vi "Get Board Information.vi"(8 "error in (no error)":errorcluster) -> (0 "error out":errorcluster, 3 "Board Information":string)   [LabVIEW 2021, in "Utilities.lvlib"]
doc: "Returns information of the application board that you connect to the NI ELVIS III workstation, such as the board ID and board status."
uses:
  <vilib>/myRIO/Instrument Drivers/Utilities/Utilities.lvlib
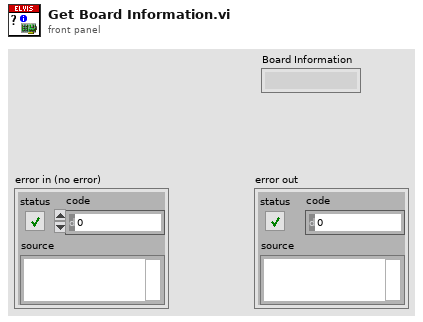
[diagram p1: front panel]
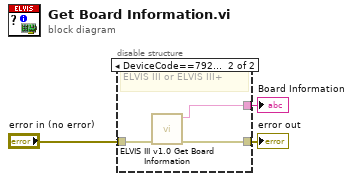
[diagram p0: block diagram]
diagram:
  n1 = disable-structure shown="DeviceCode==7928||DeviceCode==793C" {
    disable-tunnel: [w4 w7] -> w2
    disable-tunnel: "error in (no error)" -> [w4 w6]
    disable-tunnel: [_ w5] -> w1
    frame condition #0 (active) {
      # "Do nothing on other targets."
    }
    frame condition #1 {
      # "ELVIS III or ELVIS III+"
      n2 = call <vilib>:"ELVIS III v1.0 Get Board Information.vi"("error in"=w6) -> ("error out"=w7:errorcluster, "Board Information"=w5:string)  [unwired: 9 in]
    }
  }
  "error out" <- w2
  "Board Information" <- w1
